vi "Read DrivePower.vi"(8 "error in (no error)":errorcluster, 11 "DM-DriveForwardDistance in":refnum<class "DM-DriveForwardDistance.lvclass">) -> (0 "error out":errorcluster, 2 "DrivePower":dbl, 3 "DM-DriveForwardDistance out":refnum<class "DM-DriveForwardDistance.lvclass">)   [LabVIEW 2013, in "DM-DriveForwardDistance.lvclass"]
uses:
  DM-DriveForwardDistance.lvclass
  DM-DriveForwardDistance.lvclass/DM-DriveForwardDistance.ctl
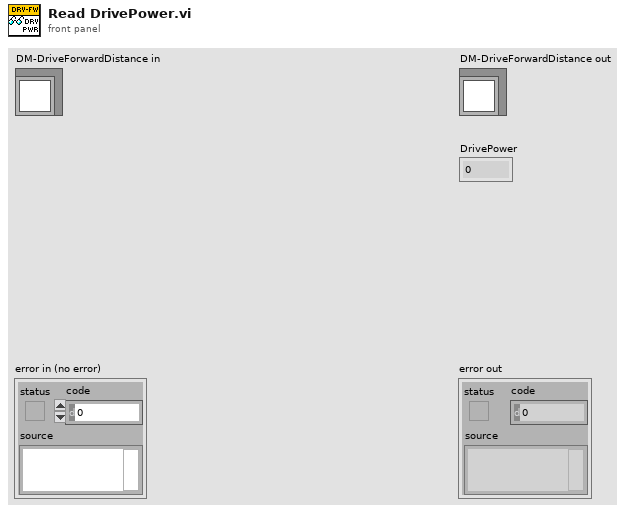
[diagram p1: front panel]
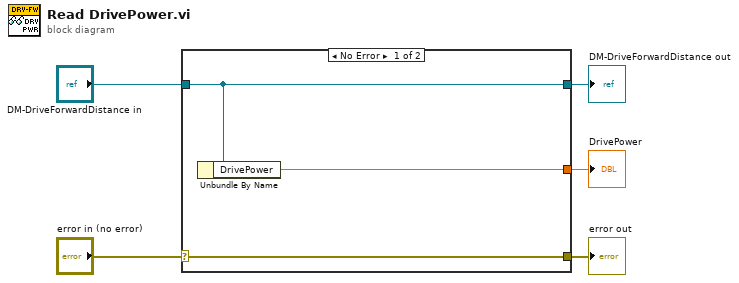
[diagram p0: block diagram]
diagram:
  n1 = case shown="No Error" "error in (no error)" {
    selector: "error in (no error)" -> [w8 w9]
    tunnel: [w8 w9] -> w4
    tunnel: [w7 w10] -> w2
    tunnel: "DM-DriveForwardDistance in" -> [w7 w10]
    tunnel: [w6 _] -> w1
    frame No Error {
      n2 = Unbundle By Name(w7) -> ("DrivePower"=w6:dbl)
    }
    frame Error {
    }
  }
  "error out" <- w4
  "DM-DriveForwardDistance out" <- w2
  "DrivePower" <- w1
